vi "Error.vi"(1 "Error con...":string, 2 "error comunicacion 2":errorcluster) -> (0 "String":string)   [LabVIEW 2015]
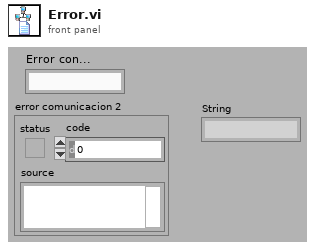
[diagram p1: front panel]
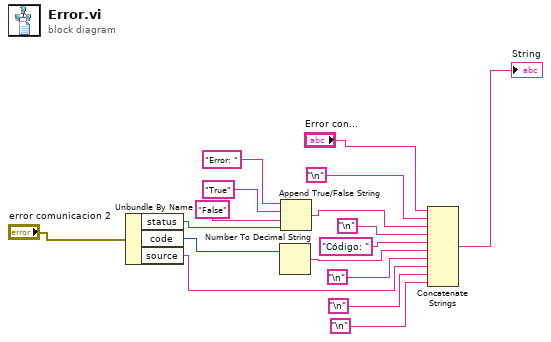
[diagram p0: block diagram]
diagram:
  n1 = Unbundle By Name("error comunicacion 2") -> ("status"=w3:bool, "code"=w7:i32, "source"=w14:string)
  n2 = Number To Decimal String(number=w7) -> (decimal integer string=w12:string)  [unwired: 1 out]
  n3 = Append True/False String(1:w3, 2:"False" ("false string"), 3:"True" ("true string"), 4:"Error: " ("string (\"\")")) -> (0:w9:string)
  n4 = Concatenate Strings("Error con...", "\n", w9, "\n", "Código: " ("string (\"\")"), w12, "\n", w14, "\n", "\n") -> (→"String":string)
